vi "Tosca-Remap Dialog.vi"(0 "Old Name In":string, 2 "Type":string, 5 "New Names":string[](array[string])) -> (4 "Old Name Out":string, 6 "New Names Out":string[](array[string]), 8 "Deleted?":bool)   [LabVIEW 2020]
panel:
  in  "New Names":u16(ring) items=["Button", "Rep Trigger", "State Change", "Trial Change"]
  in  "Message":string
  in  "Delete":bool
  in  "Replace":bool
  # "It looks like this parameter file is old or perhaps it was copied from another rig.\n\nThis dialog (and other ones like it) are trying to sort it all out.\n\nBe careful! Make sure Tosca runs as you expect. Get help if you're not sure."
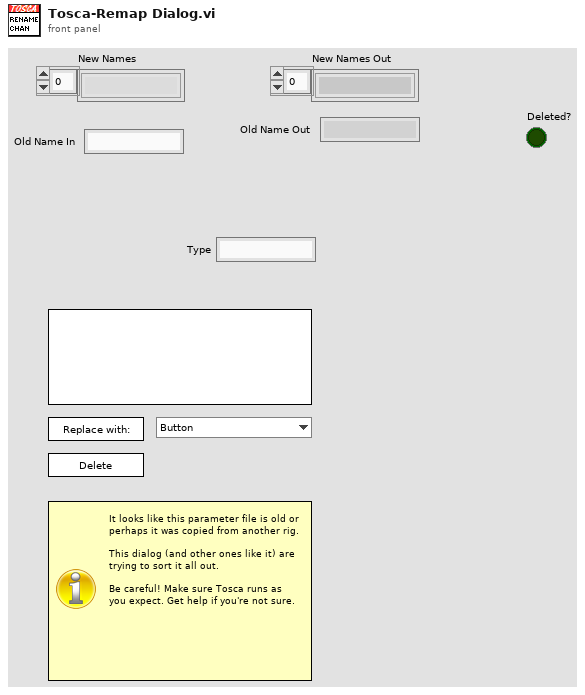
[diagram p1: front panel]
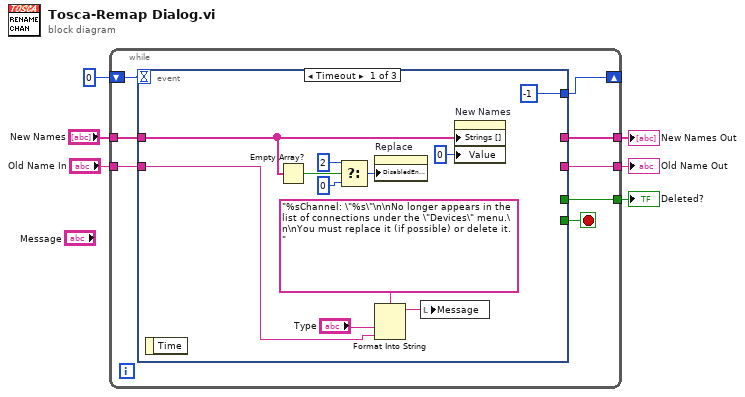
[diagram p0: block diagram]
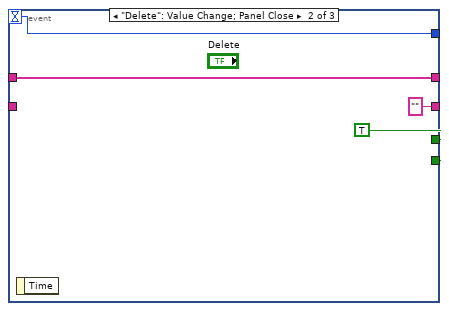
[diagram p2: hidden frame]
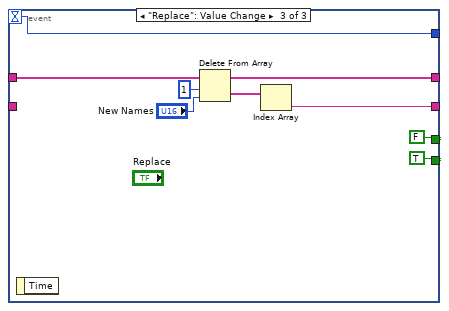
[diagram p3: hidden frame]
diagram:
  n1 = while {
    shift-right: [w13] -> _
    shift-left: 0 -> [w14]
    tunnel: "New Names" -> [w9]
    tunnel: [w12] -> w4
    tunnel: [w10] -> w3
    tunnel: "Old Name In" -> [w8]
    tunnel: [w7] -> w1
    stop <- w11 stop-if-true
    n2 = event shown="[0] Timeout" {
      selector: _ -> [_ _ _]
      dyn-events: _ -> [_ _ _]
      timeout: w14 -> [_ w29 w38]
      tunnel: [-1 w29 w38] -> w13
      tunnel: w9 -> [w20 w27 w35]
      tunnel: [_ w27 w33] -> w12
      tunnel: [_ w28 TRUE] -> w11
      tunnel: [_ w28 FALSE] -> w10
      tunnel: w8 -> [w22 _ _]
      tunnel: [_ "" ("String") w31] -> w7
      event Timeout {
        n3 = event-data() -> ()  [unwired: 1 in, 1 out]
        n4 = Empty Array?(array=w20) -> (empty?=w18:bool)
        n5 = Select(t=2, s=w18, f=0) -> (s? t:f=w19:i32)
        n6 = property on="Replace" class="Bool"("DisabledEnum"=w19) -> ()  [unwired: 2 in, 2 out]
        n7 = Format Into String(format string="%sChannel: \"%s\"\n\nNo longer appears in the list of connections under the \"Devices\" menu.\n\nYou must replace it (if possible) or delete it. ", "Type", w22) -> (resulting string=w21:string)  [unwired: 2 in, 1 out]
        n8 = local write "Message"(w21) -> ()
        n9 = property on="New Names" class="Ring (strict)"("Strings []"=w20, "Value"=0) -> ()  [unwired: 2 in, 2 out]
      }
      event "Delete": Value Change; Panel Close {
        w28 = TRUE
        n10 = event-data() -> ()  [unwired: 1 in, 1 out]
      }
      event "Replace": Value Change {
        n11 = event-data() -> ()  [unwired: 1 in, 1 out]
        n12 = Delete From Array(array=w35, length=1, index="New Names") -> (deleted portion=w32:string[], array with subset deleted=w33:string[])
        n13 = Index Array(array=w32) -> (element=w31:string)  [unwired: 1 in]
      }
    }
  }
  "New Names Out" <- w4
  "Deleted?" <- w3
  "Old Name Out" <- w1
